vi "Simple calculator.vi"() -> ()   [LabVIEW 2017]
panel:
  out "String":string
  in  "Operator":string
  out "Result":dbl
  in  "B":dbl
  in  "A":dbl
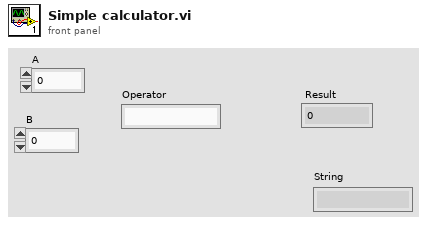
[diagram p1: front panel]
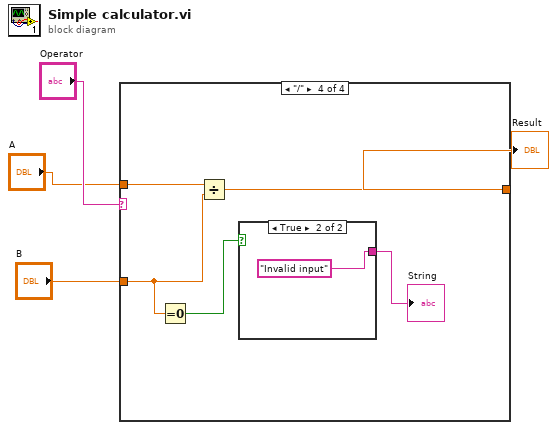
[diagram p0: block diagram]
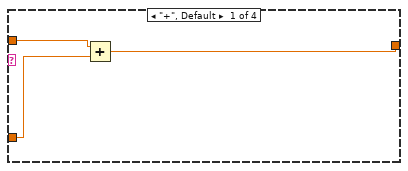
[diagram p2: hidden frame]
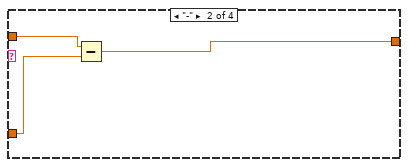
[diagram p3: hidden frame]
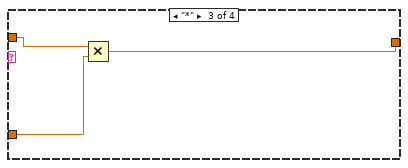
[diagram p4: hidden frame]
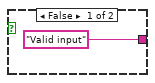
[diagram p5: hidden frame]
diagram:
  n1 = case shown="\"/\"" "Operator" {
    tunnel: "A" -> [w7 w10 w13 w18]
    tunnel: "B" -> [w6 w9 w12 w16]
    tunnel: [w5 w8 w11 w17] -> w1
    frame "+", Default {
      n2 = Add(x=w7, y=w6) -> (x+y=w5:dbl)
    }
    frame "-" {
      n3 = Subtract(x=w10, y=w9) -> (x-y=w8:dbl)
    }
    frame "*" {
      n4 = Multiply(x=w13, y=w12) -> (x*y=w11:dbl)
    }
    frame "/" {
      n5 = Equal To 0?(x=w16) -> (x = 0?=w15:bool)
      n6 = Divide(x=w18, y=w16) -> (x/y=w17:dbl)
      n7 = case shown="True" w15 {
        tunnel: ["Valid input" "Invalid input"] -> w14
        frame False {
        }
        frame True {
        }
      }
      "String" <- w14
    }
  }
  "Result" <- w1
